vi "ReadExperimentRunNode.vi"(8 "Error In":errorcluster, 11 "Experiment Run Node In":refnum<k20>) -> (0 "Error Out":errorcluster, 2 "Experiment Run":T1, 3 "Experiment Run Node Out":refnum<k20>)   [LabVIEW 2012]
uses:
  ExperimentRun.ctl
  ExperimentRunTiming.ctl
  ExperimentRunDose.ctl
  ExperimentRunFluence.ctl
  ExperimentRunTotalCharge.ctl
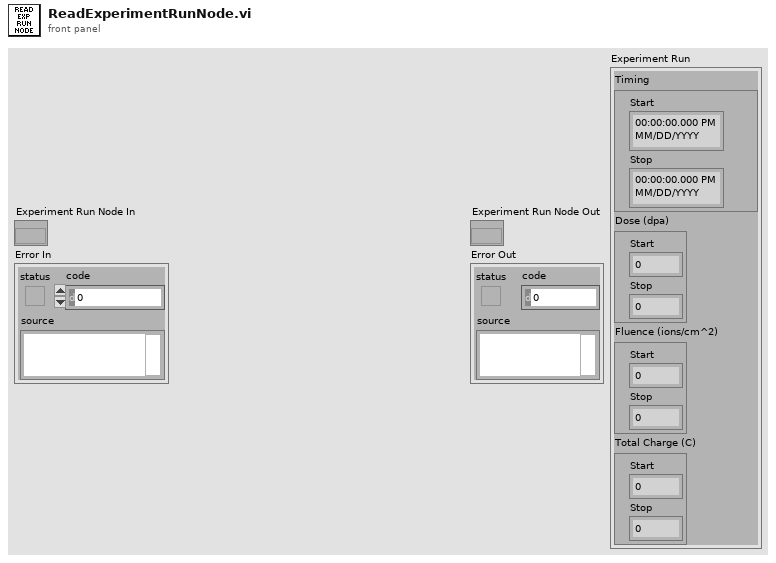
[diagram p1: front panel]
types:
  T1 = typedef "ExperimentRun.ctl" = cluster{"Timing":T2, "Dose (dpa)":T3, "Fluence (ions/cm^2)":T4, "Total Charge (C)":T5}
  T2 = typedef "ExperimentRunTiming.ctl" = cluster{"Start":timestamp, "Stop":timestamp}
  T3 = typedef "ExperimentRunDose.ctl" = cluster{"Start":dbl, "Stop":dbl}
  T4 = typedef "ExperimentRunFluence.ctl" = cluster{"Start":dbl, "Stop":dbl}
  T5 = typedef "ExperimentRunTotalCharge.ctl" = cluster{"Start":dbl, "Stop":dbl}
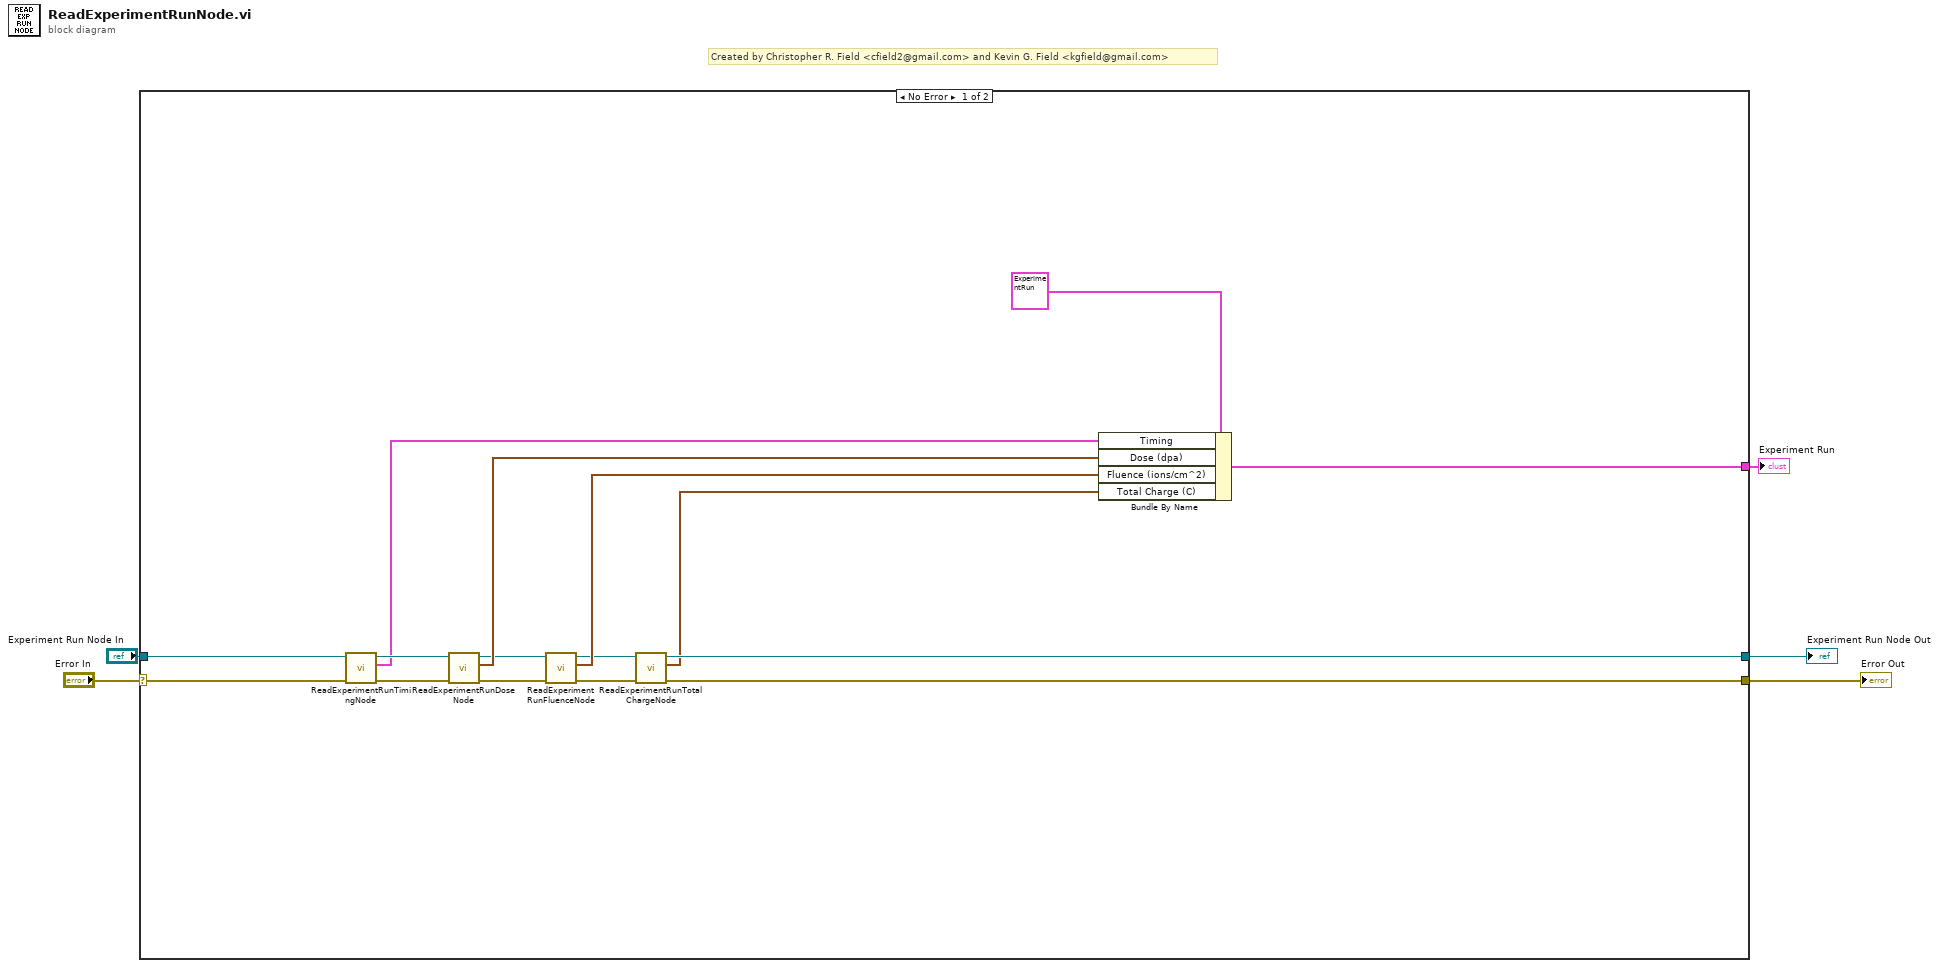
[diagram p0: block diagram]
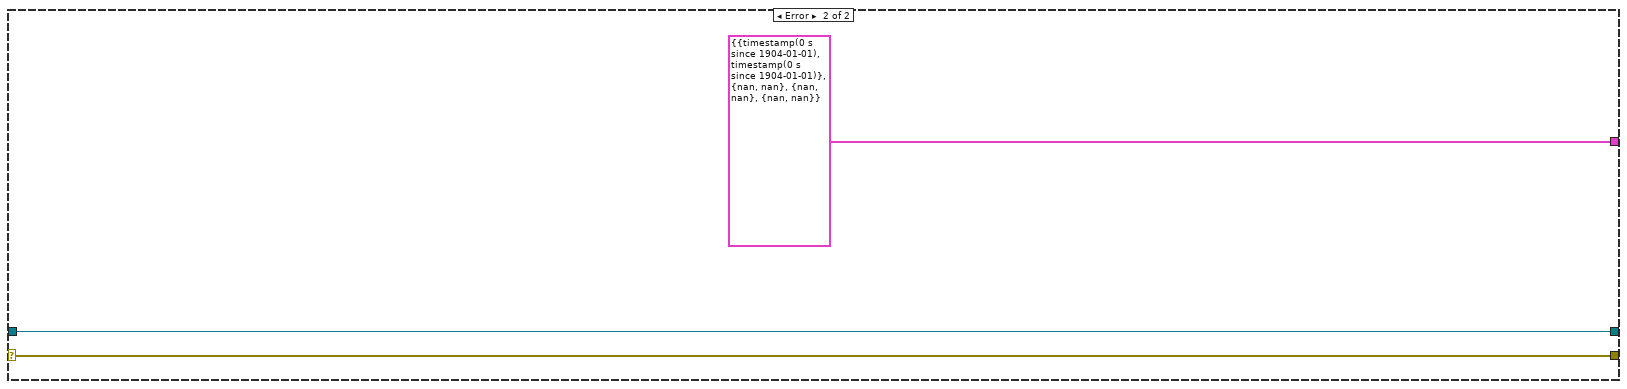
[diagram p2: hidden frame]
diagram:
  # "Created by Christopher R. Field <cfield2@gmail.com> and Kevin G. Field <kgfield@gmail.com>"
  n1 = case shown="No Error" "Error In" {
    selector: "Error In" -> [w20 w23]
    tunnel: "Experiment Run Node In" -> [w21 w24]
    tunnel: [w8 w24] -> w3
    tunnel: [w9 w23] -> w2
    tunnel: [w6 T1 {"Timing"={"Start"=timestamp(0 s since 1904-01-01), "Stop"=timestamp(0 s since 1904-01-01)}, "Dose (dpa)"={"Start"=nan, "Stop"=nan}, "Fluence (ions/cm^2)"={"Start"=nan, "Stop"=nan}, "Total Charge (C)"={"Start"=nan, "Stop"=nan}} ("Experiment Run")] -> w1
    frame No Error {
      n2 = call "ReadExperimentRunTimingNode.vi"("Error In"=w20, "Experiment Run Node In"=w21) -> ("Error Out"=w18:errorcluster, "Experiment Run Timing"=w16:T2, "Experiment Run Node Out"=w19:refnum<k20>)  [unwired: 7 in]
      n3 = call "ReadExperimentRunDoseNode.vi"("Error In"=w18, "Experiment Run Node In"=w19) -> ("Error Out"=w13:errorcluster, "Experiment Run Dose (dpa)"=w15:T3, "Experiment Run Node Out"=w14:refnum<k20>)  [unwired: 7 in]
      n4 = call "ReadExperimentRunFluenceNode.vi"("Error In"=w13, "Experiment Run Node In"=w14) -> ("Error Out"=w10:errorcluster, "Experiment Run Fluence (ions/cm^2)"=w12:T4, "Experiment Run Node Out"=w11:refnum<k20>)  [unwired: 7 in]
      n5 = call "ReadExperimentRunTotalChargeNode.vi"("Error In"=w10, "Experiment Run Node In"=w11) -> ("Error Out"=w9:errorcluster, "Experiment Run Total Charge (C)"=w7:T5, "Experiment Run Node Out"=w8:refnum<k20>)  [unwired: 7 in]
      n6 = Bundle By Name(cluster=T1 {"Timing"={"Start"=timestamp(0 s since 1904-01-01), "Stop"=timestamp(0 s since 1904-01-01)}, "Dose (dpa)"={"Start"=0.0, "Stop"=0.0}, "Fluence (ions/cm^2)"={"Start"=0.0, "Stop"=0.0}, "Total Charge (C)"={"Start"=0.0, "Stop"=0.0}} ("Experiment Run"), "Timing"=w16, "Dose (dpa)"=w15, "Fluence (ions/cm^2)"=w12, "Total Charge (C)"=w7) -> (w6:T1)
    }
    frame Error {
    }
  }
  "Experiment Run Node Out" <- w3
  "Error Out" <- w2
  "Experiment Run" <- w1
